vi "Write Notification Msg Return Info.vi"(8 "Return Priority (Normal)":T1=enum."Normal", 9 "Datum Name":string, 10 "Message Enqueuer in":refnum<class "Message Enqueuer.lvclass">, 11 "Notification Msg In":refnum<class "Notification Msg.lvclass">) -> (3 "Notification Msg Out":refnum<class "Notification Msg.lvclass">)   [LabVIEW 2020, in "ActorMessageTransport.lvlib" / "Notification Msg.lvclass"]
doc: "将返回地址信息写入通知消息。\n\n***不要覆盖此方法***\n此方法中添加了动态调度，以实现MVA框架中的向后兼容性。DD将在未来的版本中删除。"
uses:
  Notification Msg.lvclass
  <vilib>/ActorFramework/Message Enqueuer/Message Enqueuer.lvclass
  <vilib>/ActorFramework/Message Enqueuer/Message Priority.ctl
  Notification Msg.lvclass/Notification Msg.ctl
  composed-af-messages/Source/RoundTripMessage/RoundTripMessage.lvclass/RoundTripMessage.ctl
  composed-af-messages/Source/RoundTripMessage/RoundTripMessage.lvclass
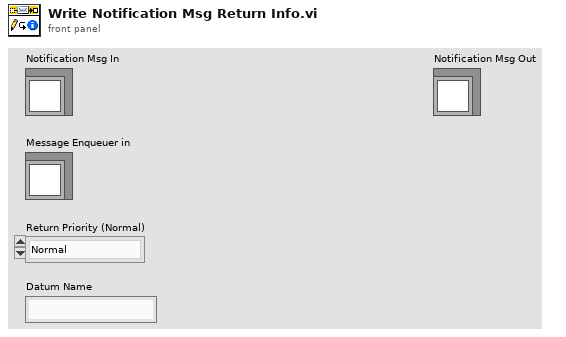
[diagram p1: front panel]
types:
  T1 = typedef "Actor Framework.lvlib/Message Enqueuer.lvclass/Message Priority.ctl" = enum16{"Low", "Normal", "High"}
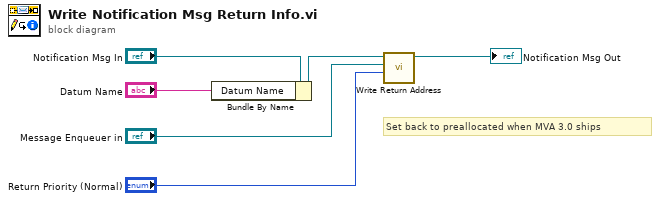
[diagram p0: block diagram]
diagram:
  # "Set back to preallocated when MVA 3.0 ships"
  n1 = Bundle By Name(cluster="Notification Msg In", "Datum Name"="Datum Name") -> (w2:refnum<class "Notification Msg.lvclass">)
  n2 = call "Write Return Address.vi"("Return Priority (Normal)"="Return Priority (Normal)", "Return Enqueuer"="Message Enqueuer in", "RoundTripMessage In"=w2) -> ("RoundTripMessage Out"=→"Notification Msg Out":refnum<class "Notification Msg.lvclass">)  [unwired: 8 in]
